vi "SmoothPath.vi"(9 "enemy_robots":T1[](array[typedef]), 10 "Path":dbl[][](array[numeric])) -> (2 "SmoothPath":dbl[][](array[numeric]))   [LabVIEW 2016]
uses:
  Core/AI Robot.ctl
  Intel/Functions Enum.ctl
  Intel/AttackerStates.ctl
panel:
  out "y":dbl
  out "x":dbl
  out "Goal":dbl[](array[numeric])
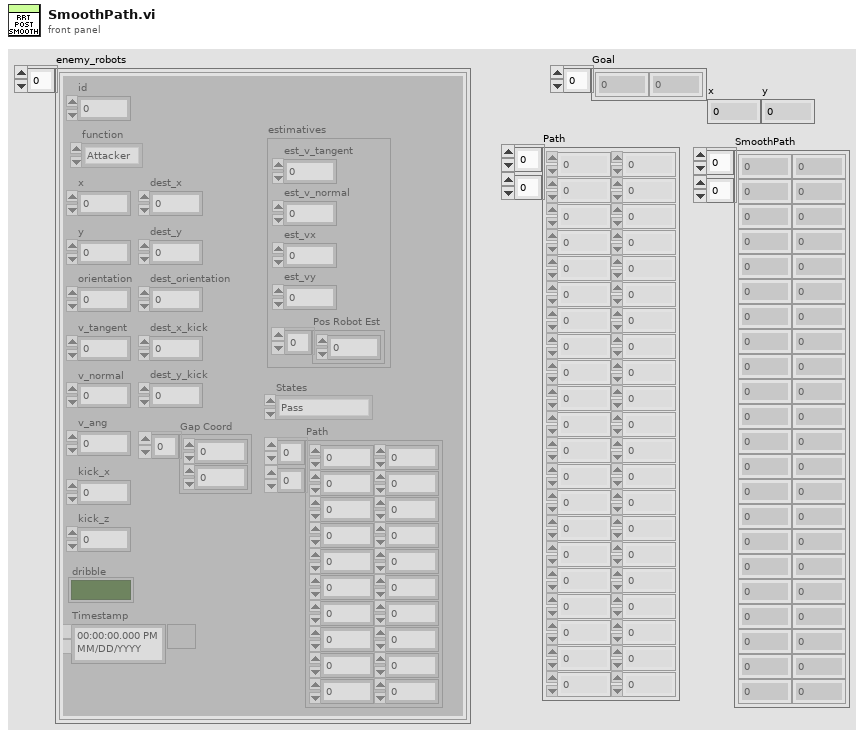
[diagram p1: front panel]
types:
  T1 = typedef "AI Robot.ctl" = cluster{"id":u32, "function":T2, "x":dbl, "y":dbl, "orientation":dbl, "v_tangent":dbl, "v_normal":dbl, "v_ang":dbl, "kick_x":dbl, "kick_z":dbl, "dribble":bool, "Timestamp":timestamp, "dest_x":dbl, "dest_y":dbl, "dest_orientation":dbl, "estimatives":cluster{"est_v_tangent":dbl, "est_v_normal":dbl, "est_vx":dbl, "est_vy":dbl, "Pos Robot Est":dbl[]}, "dest_x_kick":dbl, "dest_y_kick":dbl, "Gap Coord":dbl[], "States":T3, "Path ":dbl[][]}
  T2 = typedef "Functions Enum.ctl" = enum16{"Attacker", "Goalie", "Defender", "Striker", "Goto 0", "Dummy", "Kicker", "ZigZag"}
  T3 = typedef "AttackerStates.ctl" = enum16{"Pass", "GoToTangent", "BallGetting", "GoToKick", ""}
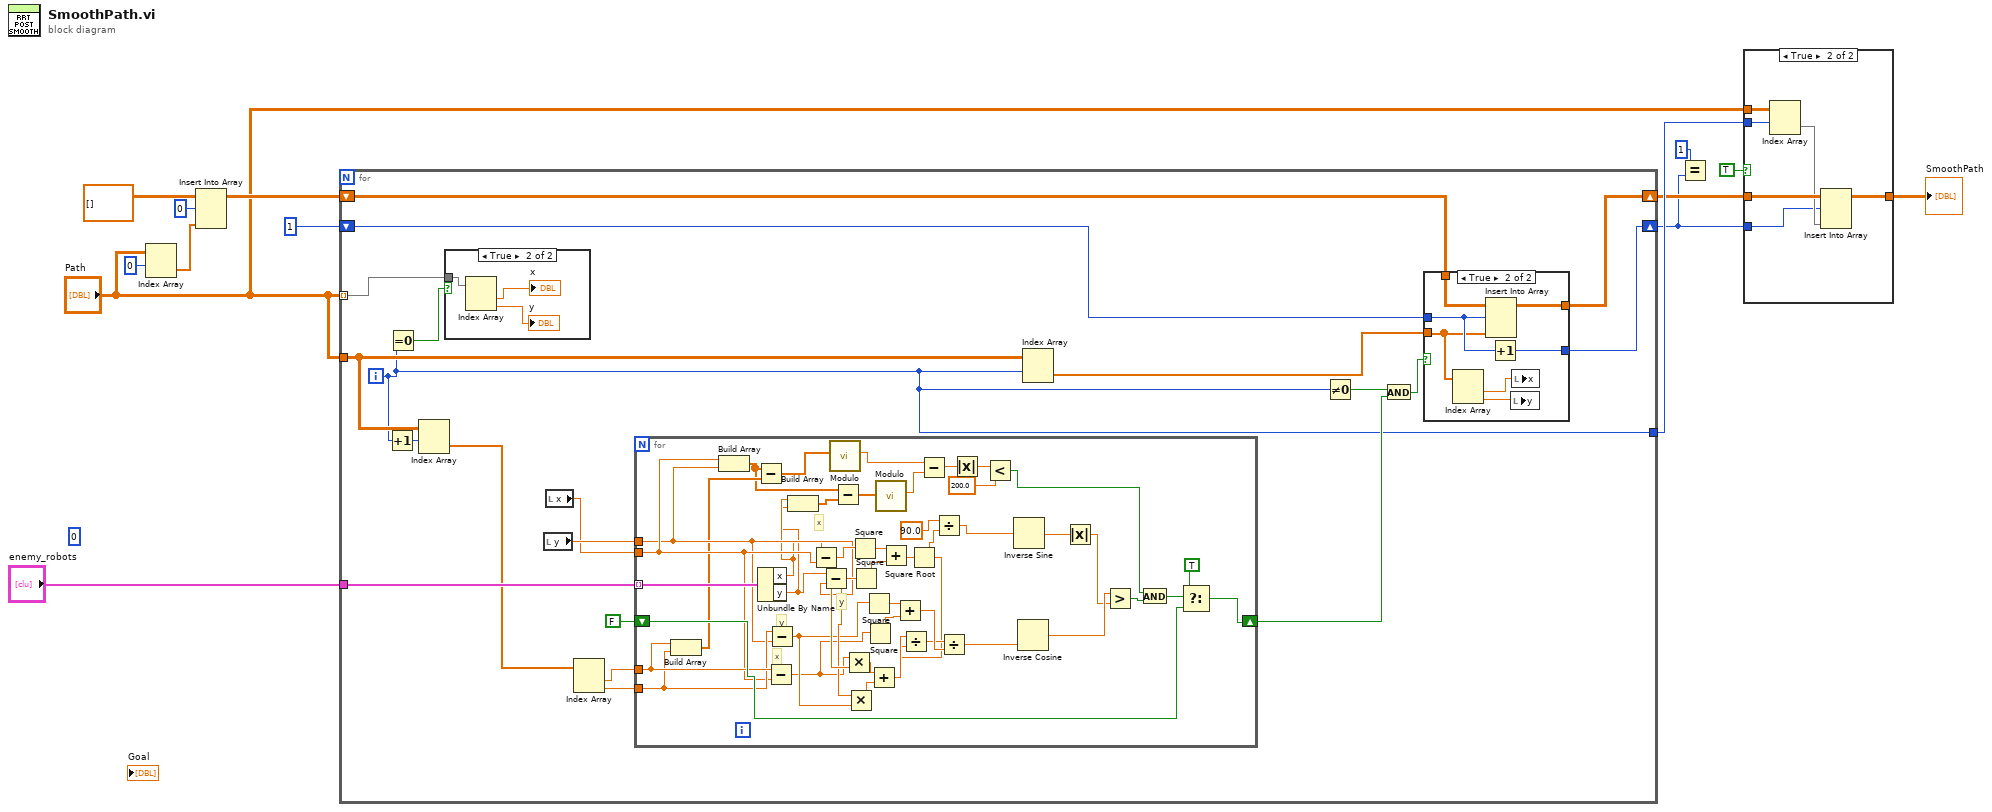
[diagram p0: block diagram]
diagram:
  (unwired) 0 ("index (row)")
  n1 = Index Array(array="Path", index (row)=0) -> (element=w11:dbl[])  [unwired: 1 in]
  n2 = Insert Into Array(array=dbl[][] [] ("Path"), index (row)=0, new element=w11) -> (w12:dbl[][])  [unwired: 1 in]
  n3 = for {
    tunnel: "Path" -> [w25] mode=indexing
    tunnel: "enemy_robots" -> [w34]
    shift-right: [w24] -> w5
    shift-left: w12 -> [w27]
    shift-right: [w23] -> w3
    shift-left: 1 ("index (row)") -> [w26]
    tunnel: "Path" -> [w21]
    tunnel: [w15] -> w6
    i -> [w15]
    n4 = Increment(x=w15) -> (x+1=w20:i32)
    n5 = Equal To 0?(x=w15) -> (x = 0?=w33:bool)
    n6 = Index Array(array=w21, index (row)=w20) -> (element=w19:dbl[])  [unwired: 1 in]
    n7 = case shown="True" w33 {
      tunnel: w25 -> [_ w46]
      frame False {
      }
      frame True {
        n8 = Index Array(array=w46) -> (element #1=→"x":dbl, element #2=→"y":dbl)  [unwired: 2 in]
      }
    }
    n9 = local read "y"() -> (w32:dbl)
    n10 = local read "x"() -> (w30:dbl)
    n11 = Index Array(array=w19) -> (element #1=w31:dbl, element #2=w29:dbl)  [unwired: 2 in]
    n12 = for {
      tunnel: w34 -> [w90] mode=indexing
      tunnel: w30 -> [w63]
      tunnel: w32 -> [w62]
      tunnel: w31 -> [w65]
      tunnel: w29 -> [w64]
      shift-right: [w70] -> w18
      shift-left: FALSE -> [w69]
      # "y"
      # "x"
      # "y"
      # "x"
      n13 = Build Array(w65, w64) -> (w61:dbl[])
      n14 = Build Array(w63, w62) -> (w57:dbl[])
      n15 = Subtract(x=w57, y=w61) -> (x-y=w60:dbl[])
      n16 = Unbundle By Name(w90) -> ("x"=w59:dbl, "y"=w58:dbl)
      n17 = Subtract(x=w65, y=w63) -> (x-y=w77:dbl)
      n18 = Subtract(x=w64, y=w62) -> (x-y=w78:dbl)
      n19 = Build Array(w59, w58) -> (w56:dbl[])
      n20 = Subtract(x=w59, y=w63) -> (x-y=w85:dbl)
      n21 = Subtract(x=w58, y=w62) -> (x-y=w84:dbl)
      n22 = call "Modulo.vi"("2D vector"=w60) -> ("Modulo"=w54:dbl)  [unwired: 10 in]
      n23 = Subtract(x=w57, y=w56) -> (x-y=w55:dbl[])
      n24 = Multiply(x=w77, y=w85) -> (x*y=w83:dbl)
      n25 = Multiply(x=w84, y=w78) -> (x*y=w82:dbl)
      n26 = Square(x=w85) -> (x^2=w89:dbl)
      n27 = Square(x=w84) -> (x^2=w88:dbl)
      n28 = Square(x=w78) -> (x^2=w80:dbl)
      n29 = Square(x=w77) -> (x^2=w79:dbl)
      n30 = Add(x=w83, y=w82) -> (x+y=w81:dbl)
      n31 = call "Modulo.vi"("2D vector"=w55) -> ("Modulo"=w53:dbl)  [unwired: 10 in]
      n32 = Add(x=w89, y=w88) -> (x+y=w87:dbl)
      n33 = Add(x=w80, y=w79) -> (x+y=w76:dbl)
      n34 = Square Root(x=w87) -> (sqrt(x)=w67:dbl)
      n35 = Divide(x=w81, y=w67) -> (x/y=w75:dbl)
      n36 = Subtract(x=w54, y=w53) -> (x-y=w52:dbl)
      n37 = Divide(x=90.0 ("y"), y=w67) -> (x/y=w86:dbl)
      n38 = Divide(x=w75, y=w76) -> (x/y=w74:dbl)
      n39 = Absolute Value(x=w52) -> (abs(x)=w51:dbl)
      n40 = Less?(x=w51, y=200.0) -> (x < y?=w47:bool)
      n41 = Inverse Sine(1:w86) -> (0:w73:dbl)
      n42 = Inverse Cosine(1:w74) -> (0:w72:dbl)
      n43 = Absolute Value(x=w73) -> (abs(x)=w71:dbl)
      n44 = Greater?(x=w72, y=w71) -> (0:w48:bool)
      n45 = And(x=w47, y=w48) -> (x .and. y?=w49:bool)
      n46 = Select(t=TRUE, s=w49, f=w69) -> (s? t:f=w70:bool)
    }
    n47 = Index Array(array=w21, index (row)=w15) -> (element=w22:dbl[])  [unwired: 1 in]
    n48 = Not Equal To 0?(x=w15) -> (x != 0?=w16:bool)
    n49 = And(x=w16, y=w18) -> (x .and. y?=w17:bool)
    n50 = case shown="True" w17 {
      tunnel: w27 -> [w36 w43]
      tunnel: w26 -> [w35 w41]
      tunnel: w22 -> [_ w39]
      tunnel: [w36 w42] -> w24
      tunnel: [w35 w40] -> w23
      frame False {
      }
      frame True {
        n51 = Index Array(array=w39) -> (element #1=w38:dbl, element #2=w37:dbl)  [unwired: 2 in]
        n52 = Insert Into Array(array=w43, index (row)=w41, new element=w39) -> (w42:dbl[][])  [unwired: 1 in]
        n53 = Increment(x=w41) -> (x+1=w40:i32)
        n54 = local write "y"(w37) -> ()
        n55 = local write "x"(w38) -> ()
      }
    }
  }
  n56 = Equal?(x=1, y=w3) -> ()  [unwired: 1 out]
  n57 = case shown="True" TRUE {
    tunnel: "Path" -> [_ w97]
    tunnel: w6 -> [_ w96]
    tunnel: w5 -> [w91 w95]
    tunnel: [w91 w94] -> w4
    tunnel: w3 -> [_ w92]
    frame False {
    }
    frame True {
      n58 = Index Array(array=w97, index (row)=w96) -> (element=w93:dbl[])  [unwired: 1 in]
      n59 = Insert Into Array(array=w95, index (row)=w92, new element=w93) -> (w94:dbl[][])  [unwired: 1 in]
    }
  }
  "SmoothPath" <- w4
